vi "扫码页面.vi"(2 "Barcode 输入":string caption="扫描条码/Barcode") -> (0 "Return":string)   [LabVIEW 2015]
panel:
  in  "长度控制":u32=24
  out "实际长度":i32
  in  "Barcode":string caption="扫描条码/Barcode"
  in  "Exit":bool
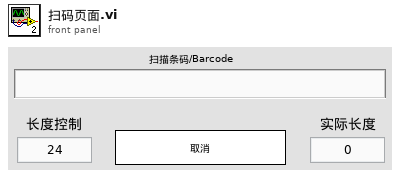
[diagram p1: front panel]
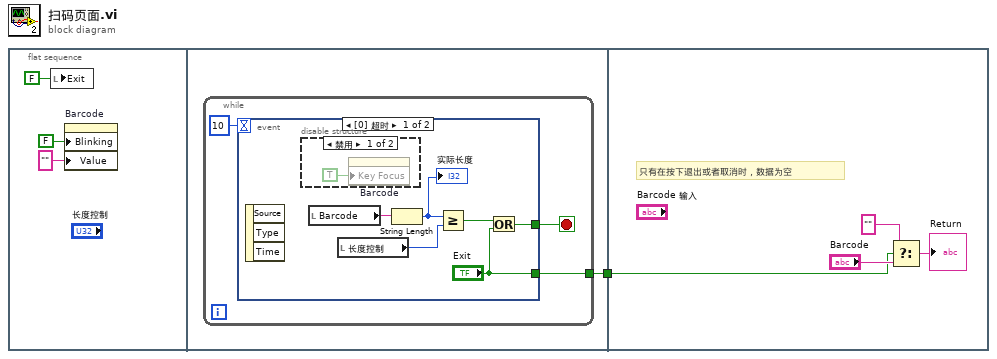
[diagram p0: block diagram]
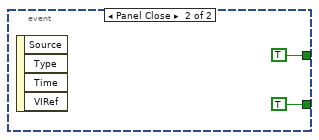
[diagram p3: hidden frame]
diagram:
  n1 = flat-sequence {
    tunnel: [w5] -> w1
    tunnel: w1 -> [w19]
    frame #0 {
      n2 = local write "Exit"(FALSE ("Exit")) -> ()
      n3 = property on="Barcode" class="Str"("Blinking"=FALSE, "Value"="" ("Barcode")) -> ()  [unwired: 2 in, 2 out]
    }
    frame #1 {
      n4 = while {
        tunnel: [w7] -> w5
        stop <- w8 stop-if-true
        n5 = event shown="[0] 超时" {
          selector: _ -> [_ _]
          dyn-events: _ -> [_ _]
          timeout: 10 -> [_ _]
          tunnel: [w14 TRUE] -> w8
          tunnel: ["Exit" TRUE ("Exit")] -> w7
          event Timeout {
            n6 = event-data() -> ()  [unwired: 1 in, 3 out]
            n7 = disable-structure shown="禁用" {
              frame Disabled {
                n8 = property on="Barcode" class="Str"("Key Focus"=TRUE ("键选中")) -> ()  [unwired: 2 in, 2 out]
              }
              frame Enabled {
              }
            }
            n9 = local read "Barcode"() -> (w12:string)
            n10 = local read "长度控制"() -> (w9:u32)
            n11 = String Length(string=w12) -> (length=w10:i32)
            "实际长度" <- w10
            n12 = Greater Or Equal?(x=w10, y=w9) -> (x >= y?=w11:bool)
            n13 = Or(x=w11, y="Exit") -> (x .or. y?=w14:bool)
          }
          event Panel Close {
            n14 = event-data() -> ()  [unwired: 1 in, 4 out]
          }
        }
      }
    }
    frame #2 {
      # "只有在按下退出或者取消时，数据为空"
      n15 = Select(t="", s=w19, f="Barcode") -> (s? t:f=→"Return":string)
    }
  }
